vi "NewGame.vi"(7 "PongType (ChildObject)":refnum<class "Pong.lvclass">, 8 "error in (no error)":errorcluster, 11 "FPGA_ref":T1) -> (0 "error out":errorcluster, 3 "Pong out":refnum<class "Pong.lvclass">)   [LabVIEW 2019, in "RT_Game.lvlib" / "Pong.lvclass"]
uses:
  Pong.lvclass
  C:/Users/FreshBob/Dropbox/VIs/myRIO_GameConsole/RT/RT_Game/Game/Game.lvclass
  FPGA_Interface.ctl
  Game/Coordinate.ctl
  PongBall/PongBall.lvclass
  C:/Users/FreshBob/Dropbox/VIs/myRIO_GameConsole/RT/RT_Game/RT_Sprite/RT_Sprite.lvclass
  TileTime/TileTimer.lvclass
  C:/Users/FreshBob/Dropbox/VIs/myRIO_GameConsole/RT/RT_Game/GameObject/GameObject.lvclass
  TileTime/TileTimer.lvclass/TileTimer.ctl
  GameObject/GameObject.lvclass/GameObject.ctl
  Pong.lvclass/Pong.ctl
  PongPanel/PongPanel.lvclass/PongPanel.ctl
  Game/Game.lvclass/Game.ctl
  TileTime/Write StartTime.vi
  GameObject/Write position.vi
  PongPanel/Write StartPos.vi
  PongPanel/Write limit_y.vi
  PongPanel/Write Speed.vi
  GameObject/Write IsActive.vi
  PongPanel/Write limit_x_down.vi
  PongPanel/Write limit_x_up.vi
  PongPanel/Write limit_y_down.vi
  Game/Read Singleplayer.vi
  Game/Write Sprites.vi
  PongPanel/PongPanel.lvclass
  Game/Game.lvclass
  RT_Sprite/RT_Sprite.lvclass
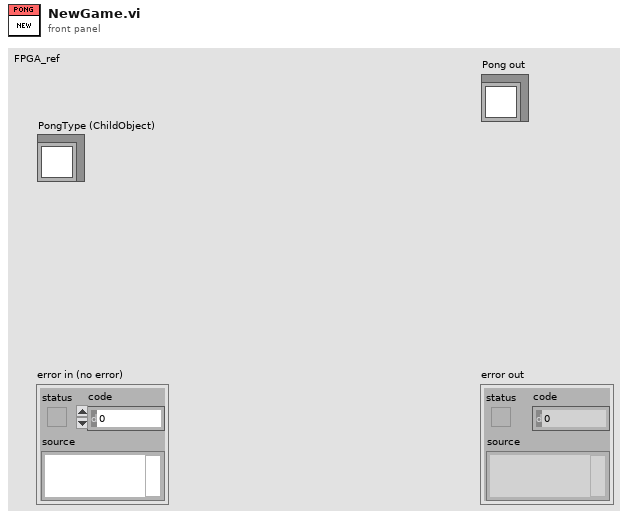
[diagram p1: front panel]
types:
  T1 = typedef "FPGA_Interface.ctl" = refnum<k20>
  T2 = typedef "RT_Game.lvlib/Game.lvclass/Coordinate.ctl" = cluster{"x":dbl, "y":dbl}
  T3 = cluster{"left_panel":refnum<class "PongPanel.lvclass">, "right_panel":refnum<class "PongPanel.lvclass">, "ball":refnum<class "PongBall.lvclass">}
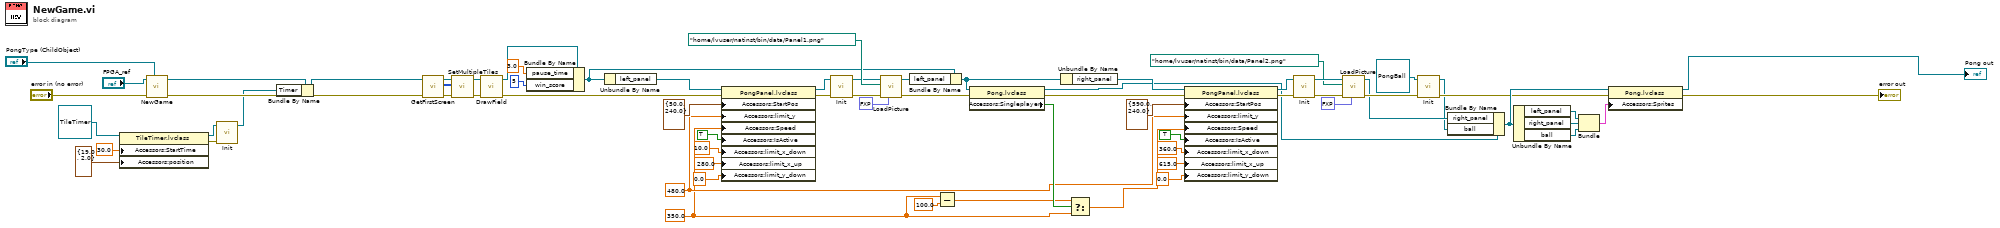
[diagram p0: block diagram]
diagram:
  w11 = 350.0 ("Speed")
  w12 = 480.0 ("Limit")
  n1 = property class="TileTimer.lvclass"(reference=refnum<class "TileTimer.lvclass"> refnum ("Timer"), "Accessors:StartTime"=30.0 ("StartTime"), "Accessors:position"=T2 {"x"=19.0, "y"=2.0} ("position")) -> (reference out=w5:refnum<class "TileTimer.lvclass">, error out=w8:errorcluster)  [unwired: 1 in]
  n2 = call-parent "NewGame.vi"("GameType (ChildObject)"="PongType (ChildObject)", "error in (no error)"="error in (no error)", "FPGA_ref"="FPGA_ref") -> ("error out"=w38:errorcluster, "Game out"=w24:refnum<class "Pong.lvclass">)  [unwired: 7 in]
  n3 = call-dynamic "Init.vi"("error in (no error)"=w8, "TileTimer in"=w5) -> ("TileTimer out"=w1:refnum<class "TileTimer.lvclass">)  [unwired: 8 in, 1 out]
  n4 = Bundle By Name(cluster=w24, "Timer"=w1) -> (w2:refnum<class "Pong.lvclass">)
  n5 = call-dynamic "GetFirstScreen.vi"("error in (no error)"=w38, "Pong in"=w2) -> ("error out"=w25:errorcluster, "Array"=w22:u32[][], "Pong out"=w23:refnum<class "Pong.lvclass">)  [unwired: 7 in]
  n6 = call "SetMultipleTiles.vi"("error in (no error)"=w25, "TileCodes"=w22, "Game in"=w23) -> ("error out"=w26:errorcluster, "Game out"=w20:refnum<class "Pong.lvclass">)  [unwired: 7 in]
  n7 = call "DrawField.vi"("error in (no error)"=w26, "Pong in"=w20) -> ("error out"=w21:errorcluster, "Pong out"=w19:refnum<class "Pong.lvclass">)  [unwired: 8 in]
  n8 = Bundle By Name(cluster=w19, "pause_time"=3.0, "win_score"=i16 5) -> (w13:refnum<class "Pong.lvclass">)
  n9 = Unbundle By Name(w13) -> ("left_panel"=w66:refnum<class "PongPanel.lvclass">)
  n10 = property class="PongPanel.lvclass"(reference=w66, error in=w21, "Accessors:StartPos"=T2 {"x"=50.0, "y"=240.0} ("Position"), "Accessors:limit_y"=w12, "Accessors:Speed"=w11, "Accessors:IsActive"=TRUE ("IsActive"), "Accessors:limit_x_down"=10.0 ("limit_x_down"), "Accessors:limit_x_up"=280.0 ("limit_x_up"), "Accessors:limit_y_down"=0.0 ("limit_y_down")) -> (reference out=w40:refnum<class "PongPanel.lvclass">, error out=w64:errorcluster)
  n11 = call-dynamic "Init.vi"("error in (no error)"=w64, "PongPanel in"=w40) -> ("error out"=w41:errorcluster, "PongPanel out"=w39:refnum<class "PongPanel.lvclass">)  [unwired: 8 in]
  n12 = call "LoadPicture.vi"("Transparent Color"=fxp<+,3,3> 4.0, "error in (no error)"=w41, "Picture Path"=path "/home/lvuser/natinst/bin/data/Panel1.png" ("ImagePath"), "RT_Sprite in"=w39) -> ("error out"=w48:errorcluster, "RT_Sprite out"=w47:refnum<class "PongPanel.lvclass">)  [unwired: 6 in]
  n13 = Bundle By Name(cluster=w13, "left_panel"=w47) -> (w17:refnum<class "Pong.lvclass">)
  n14 = Subtract(x=w11, y=100.0 ("x")) -> (x-y=w10:dbl)
  n15 = property class="Pong.lvclass"(reference=w17, error in=w48) -> (reference out=w15:refnum<class "Pong.lvclass">, error out=w18:errorcluster, "Accessors:Singleplayer"=w16:bool)
  n16 = Unbundle By Name(w17) -> ("right_panel"=w65:refnum<class "PongPanel.lvclass">)
  n17 = Select(t=w10, s=w16, f=w11) -> (s? t:f=w30:dbl)
  n18 = property class="PongPanel.lvclass"(reference=w65, error in=w18, "Accessors:StartPos"=T2 {"x"=590.0, "y"=240.0} ("Position"), "Accessors:limit_y"=w12, "Accessors:Speed"=w30, "Accessors:IsActive"=TRUE ("IsActive"), "Accessors:limit_x_down"=360.0 ("limit_x_down"), "Accessors:limit_x_up"=615.0 ("limit_x_up"), "Accessors:limit_y_down"=0.0 ("limit_y_down")) -> (reference out=w43:refnum<class "PongPanel.lvclass">, error out=w63:errorcluster)
  n19 = call-dynamic "Init.vi"("error in (no error)"=w63, "PongPanel in"=w43) -> ("error out"=w44:errorcluster, "PongPanel out"=w42:refnum<class "PongPanel.lvclass">)  [unwired: 8 in]
  n20 = call "LoadPicture.vi"("Transparent Color"=fxp<+,3,3> 4.0, "error in (no error)"=w44, "Picture Path"=path "/home/lvuser/natinst/bin/data/Panel2.png" ("ImagePath"), "RT_Sprite in"=w42) -> ("error out"=w50:errorcluster, "RT_Sprite out"=w49:refnum<class "PongPanel.lvclass">)  [unwired: 6 in]
  n21 = call-dynamic "Init.vi"("error in (no error)"=w50, "PongBall in"=refnum<class "PongBall.lvclass"> refnum ("RT_Game.lvlib:PongBall.lvclass")) -> ("error out"=w46:errorcluster, "PongBall out"=w14:refnum<class "PongBall.lvclass">)  [unwired: 8 in]
  n22 = Bundle By Name(cluster=w15, "right_panel"=w49, "ball"=w14) -> (w57:refnum<class "Pong.lvclass">)
  n23 = Unbundle By Name(w57) -> ("left_panel"=w56:refnum<class "PongPanel.lvclass">, "right_panel"=w55:refnum<class "PongPanel.lvclass">, "ball"=w52:refnum<class "PongBall.lvclass">)
  n24 = Bundle("left_panel"=w56, "right_panel"=w55, "ball"=w52) -> (w51:T3)  [unwired: 1 in]
  n25 = property class="Pong.lvclass"(reference=w57, error in=w46, "Accessors:Sprites"=w51) -> (reference out=→"Pong out":refnum<class "Pong.lvclass">, error out=→"error out":errorcluster)
